vi "LabView - Control Motors Duty Cycle and direction using LabView Arduino Firmware and L293D.vi"() -> ()   [LabVIEW 2022 SP3]
uses:
  <vilib>/MakerHub/LINX/Public/Peripherals/Digital/Digital Write N Chans.vi
  <vilib>/MakerHub/LINX/Public/Peripherals/Digital/Digital Read N Chans.vi
  <vilib>/MakerHub/LINX/Private/Local IO/LinxDigitalWrite.vi
  <vilib>/MakerHub/LINX/Public/Utilities/Check Channel.vi
  <vilib>/MakerHub/LINX/Private/Local IO/LinxDigitalRead.vi
  <vilib>/MakerHub/LINX/Public/Utilities/Open Serial.vi
  <vilib>/MakerHub/LINX/Public/Peripherals/PWM/PWM Set Duty Cycle N Chans.vi
  <vilib>/MakerHub/LINX/Private/Utilties/Generate Error.vi
  <vilib>/MakerHub/LINX/LMH-LINX.lvlib
panel:
  in  "DI Channels":u8[](array[numeric])
  in  "DO Channels":u8[](array[numeric])
  in  "PWM Channels":u8[](array[numeric])
  out "IR LED":bool[](array[boolean])
  in  "Duty Cycle":dbl(slide) scale=0.0..1.0
  in  "Motor Directions (Input)":bool[](array[boolean])
  in  "stop":bool
  in  "Serial Port":refnum<visa-resource-name>="N/A"
  # "Control Unit"
  # "Channels Data"
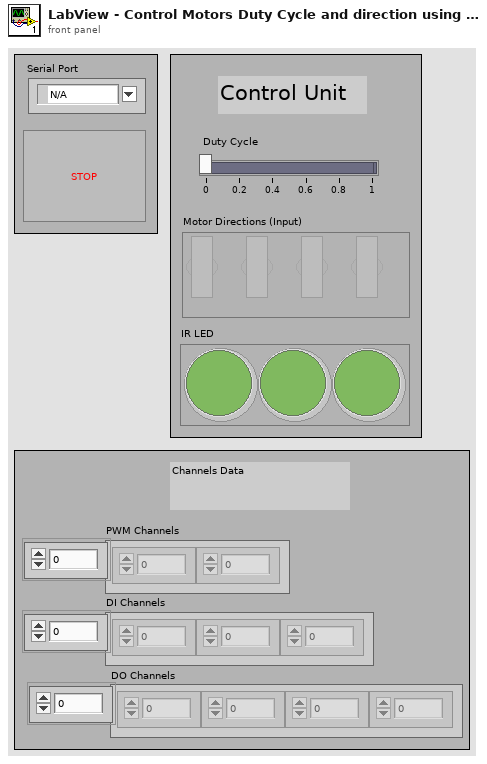
[diagram p1: front panel]
types:
  T1 = typedef "LMH-LINX.lvlib/LINX Ref.ctl" = cluster{"IO":T2, "Interface":T3, "LINX Device Config":T4}
  T2 = typedef "LMH-LINX.lvlib/Platform.ctl" = enum16{"Remote", "Local"}
  T3 = typedef "LMH-LINX.lvlib/Interface.ctl" = enum16{"Serial", "TCP"}
  T4 = typedef "LMH-LINX.lvlib/Device.lvlib/LINX Device Config.ctl" = cluster{"Interface":T3, "COM Port":refnum<visa-resource-name>, "TCP Configuration":T5, "Device Family":u8, "Device ID":u8, "Device Name":string, "TCP Ref":refnum<k5>, "Channels":T6}
  T5 = typedef "LMH-LINX.lvlib/Device.lvlib/TCP Config.ctl" = cluster{"IP Address":string, "Port":u16}
  T6 = typedef "LMH-LINX.lvlib/Channels.ctl" = cluster{"DI":u8[], "DO":u8[], "AI":u8[], "AO":u8[], "PWM":u8[], "QE":u8[], "UART":u8[], "I2C 2":u8[], "SPI":u8[], "CAN":u8[], "Servo":u8[], "AI Ref (V)":dbl, "AI Resolution (Bits)":u8, "AO Ref (V)":dbl, "AO Resolution (Bits)":u8}
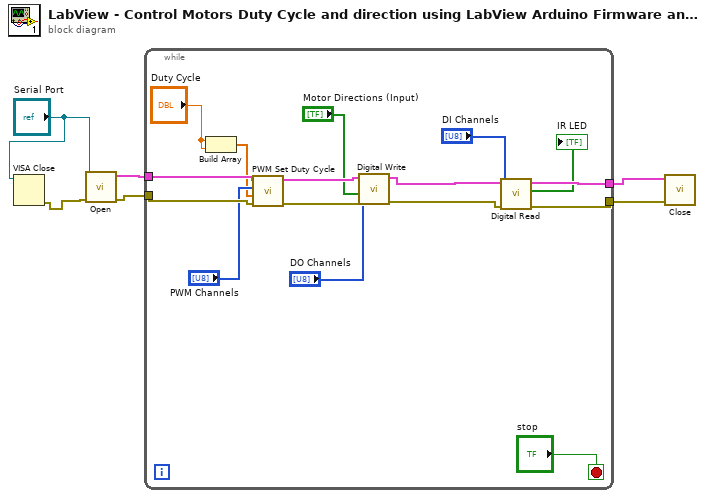
[diagram p0: block diagram]
diagram:
  n1 = VISA Close(VISA resource name="Serial Port") -> (error out=w6:errorcluster)  [unwired: 1 in]
  n2 = call-poly <vilib>:"Open.vi"("Error In"=w6, "Serial Port"="Serial Port") -> ("Error Out"=w3:errorcluster, "LINX Resource"=w4:T1)  [unwired: 7 in, 1 out]
  n3 = while {
    tunnel: w4 -> [w22]
    tunnel: w3 -> [w20]
    tunnel: [w13] -> w2
    tunnel: [w11] -> w1
    stop <- "stop" stop-if-true
    n4 = Build Array("Duty Cycle", "Duty Cycle") -> (w7:dbl[])
    n5 = call-poly <vilib>:"PWM Set Duty Cycle.vi"("Error In"=w20, "Duty Cycles"=w7, "PWM Channels"="PWM Channels", "LINX Resource"=w22) -> ("Error Out"=w19:errorcluster, "LINX Resource"=w21:T1)  [unwired: 6 in]
    n6 = call-poly <vilib>:"Digital Write.vi"("Error In"=w19, "Values"="Motor Directions (Input)", "DO Channels"="DO Channels", "LINX Resource"=w21) -> ("Error Out"=w12:errorcluster, "LINX Resource"=w14:T1)  [unwired: 6 in]
    n7 = call-poly <vilib>:"Digital Read.vi"("Error In"=w12, "DI Channels"="DI Channels", "LINX Resource"=w14) -> ("Error Out"=w11:errorcluster, "Values"=→"IR LED":bool[], "LINX Resource"=w13:T1)  [unwired: 6 in]
  }
  n8 = call <vilib>:"Close.vi"("Error In"=w1, "LINX Resource"=w2) -> ()  [unwired: 9 in, 1 out]
